vi "CreateMethod.vi"(0 "LibWriter":refnum<class "LibWriter.lvclass">, 1 "ClassItemRefIn":refnum<vi>, 2 "CreateMethodData":T1={"MethodName"="", "RelativeMethodPath"=path "", "MethodDescription"="", "Scope/Visibility"=enum."Use Parent Folder Scope", "MethodTemplateName"="", "IconOut"=[], "RelativeProjectLibPath"="", "OpenViAfterCreation"=FALSE, "ExtraCreateParameters"=variant, "IconDetails"={"IconSize"=enum."1 c-term high", "ImageRows(32)"=32, "ConnectorPaneHeight"=[]}, "AF-Option"=variant, "TemplatePath"=path ""} {"IconOut" format="%x"}, 5 "error in (no error)":errorcluster) -> (14 "LibWriter":refnum<class "LibWriter.lvclass">, 15 "ClassItemRefOut":refnum<vi>, 16 "MethodPaths":path[](array[path]), 19 "error out":errorcluster)   [LabVIEW 2014, in "LibWriter.lvclass"]
uses:
  <resource>/Framework/Providers/Open_GDS/ClassProviders/LibProvider_BaseClassInterface/LibWriter_class/ClassWriter_class/LibWriter.lvclass
  <resource>/Framework/Providers/Open_GDS/ClassProviders/LibProvider_BaseClassInterface/LibWriter_class/CreateMethodData.ctl
  <resource>/Framework/Providers/Open_GDS/ClassProviders/Provider_EndevoGOOP300/GOOP300_SubVIs/GOOP300_MethodScopeType.ctl
  <resource>/Framework/Providers/Open_GDS/ClassProviders/Provider_LvNativeClass/ClassWriterNative_class/IconDetails.ctl
  <resource>/Framework/Providers/Open_GDS/ClassProviders/Provider_LvNativeClass/ClassWriterNative_class/IconSize.ctl
  <resource>/Framework/Providers/Open_GDS/ClassProviders/Provider_LvNativeClass/ClassWriterNative_class/ClassWriterNative.lvclass
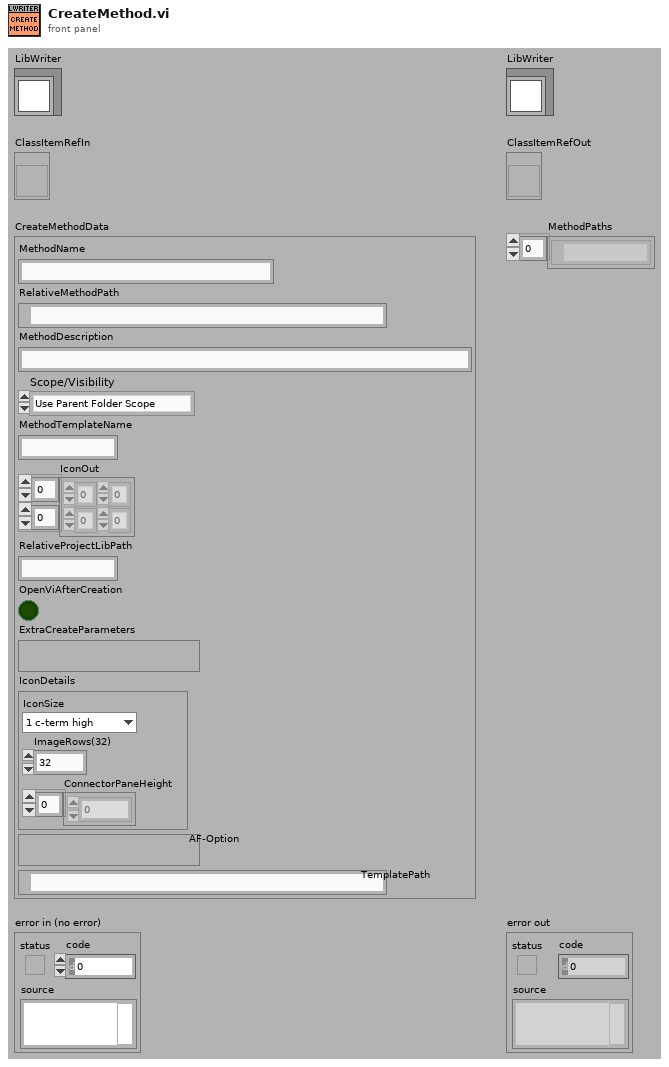
[diagram p1: front panel]
types:
  T1 = typedef "LibWriter.lvclass/CreateMethodData.ctl" = cluster{"MethodName":string, "RelativeMethodPath":path, "MethodDescription":string, "Scope/Visibility":T2, "MethodTemplateName":string, "IconOut":u8[][], "RelativeProjectLibPath":string, "OpenViAfterCreation":bool, "ExtraCreateParameters":variant, "IconDetails":T3, "AF-Option":variant, "TemplatePath":path}
  T2 = typedef "GOOP300_MethodScopeType.ctl" = enum16{"Use Parent Folder Scope", "Public", "Protected", "Private", "Community"}
  T3 = typedef "ClassWriterNative.lvclass/IconDetails.ctl" = cluster{"IconSize":T4, "ImageRows(32)":i32, "ConnectorPaneHeight":i32[]}
  T4 = typedef "ClassWriterNative.lvclass/IconSize.ctl" = enum16{"Full", "1 c-term high", "2 c-term high", "3 c-term high"}
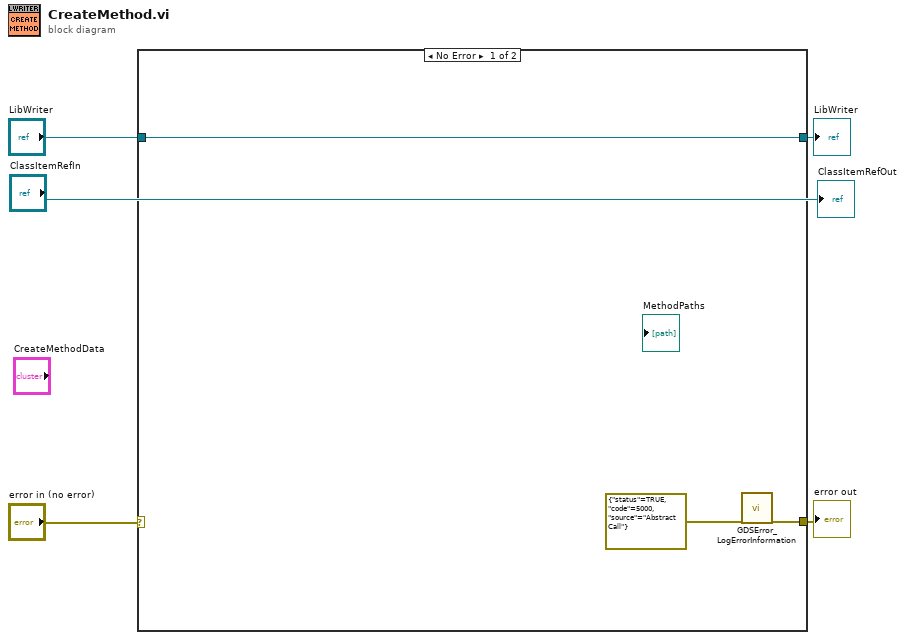
[diagram p0: block diagram]
diagram:
  n1 = case shown="No Error" "error in (no error)" {
    selector: "error in (no error)" -> [_ w9]
    tunnel: "LibWriter" -> [w8 w10]
    tunnel: [w6 w9] -> w4
    tunnel: [w8 w10] -> w3
    frame No Error {
      n2 = call <resource>:"GDSError_LogErrorInformation.vi"("error in (no error)"=errorcluster {"status"=TRUE, "code"=5000, "source"="Abstract Call"} ("error IO")) -> ("error out"=w6:errorcluster)  [unwired: 18 in]
    }
    frame Error {
    }
  }
  "LibWriter" <- w3
  "error out" <- w4
  "ClassItemRefOut" <- "ClassItemRefIn"
